vi "Write CustomCanon.vi"(8 "error in (no error)":errorcluster, 10 "CustomCanon":string, 11 "Canon in":refnum<class "Canon.lvclass">) -> (0 "error out":errorcluster, 3 "Canon out":refnum<class "Canon.lvclass">)   [LabVIEW 2021, in "Canon.lvclass"]
uses:
  Canon.lvclass
  Canon.lvclass/Canon.ctl
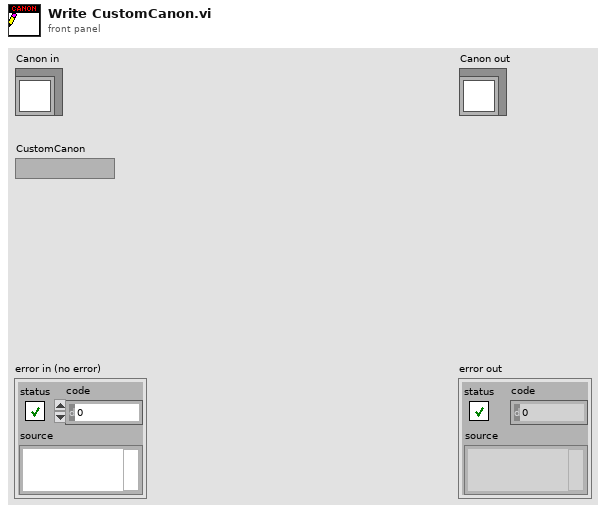
[diagram p1: front panel]
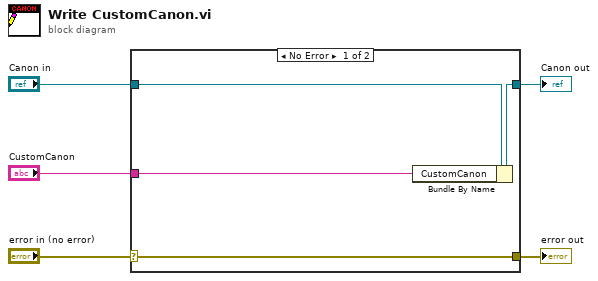
[diagram p0: block diagram]
diagram:
  n1 = case shown="No Error" "error in (no error)" {
    selector: "error in (no error)" -> [w9 w10]
    tunnel: [w9 w10] -> w4
    tunnel: [w7 w11] -> w2
    tunnel: "Canon in" -> [w8 w11]
    tunnel: "CustomCanon" -> [w6 _]
    frame No Error {
      n2 = Bundle By Name(cluster=w8, "CustomCanon"=w6) -> (w7:refnum<class "Canon.lvclass">)
    }
    frame Error {
    }
  }
  "error out" <- w4
  "Canon out" <- w2
